vi "TEST-Main.vi"() -> ()   [LabVIEW 2020, in "CSMStand(Lite)-test.lvlib"]
doc: "------------- lvcsm -------------\n[CSMStates]\nItem 0 = \"Event Structure\"\nItem 1 = \"Idle\"\nItem 2 = \"CSM Documentation\"\nItem 3 = \"Error Handler\"\nItem 4 = \"VI Reference\"\nItem 5 = \"Critical Error\"\nItem 6 = \"Target Timeout Error\"\nItem 7 = \"Target Error\"\nItem 8 = \"Async Response\"\nItem 9 = \"Response\"\nItem 10 = \"Async Message Posted\"\nItem 11 = \"Initialize Core Data\"\nItem 12 = \"Exit\"\nItem 13 = \"Data: Initialize\"\nItem 14 = \"Data: Cleanup\"\nItem 15 = \"Events: Register\"\nItem 16 = \"Events: Unregister\"\nItem 17 = \"UI: Initialize\"\nItem 18 = \"UI: Cursor Set\"\nItem 19 = \"UI: Front Panel State\"\nItem 20 = \"Macro: Initialize\"\nItem 21 = \"Macro: Exit\"\nItem 22 = \"API: API1\"\nItem 23 = \"API: API2\"\nItem 24 = \"Internal: action1\"\nItem 25 = \"Internal: action2\"\n\n[CSMStatus]\nItem 0 = \"Error Occurred@Error Handler\""
uses:
  <vilib>/numeric/Random Number (Range) DBL.vi
  510b3246-460f-4579-b188-a02bea6833a2.vi
  <userlib>/_NEVSTOP/Communicable State Machine(CSM)/_Support/Common/Format Timestamp.vi
  <userlib>/_NEVSTOP/Communicable State Machine(CSM)/AdvanceAPI/CSM - Keywords.vi
  <userlib>/_NEVSTOP/Communicable State Machine(CSM)/AdvanceAPI/CSM - Revert Arguments-Safe String.vi
  <userlib>/_NEVSTOP/Communicable State Machine(CSM)/AdvanceAPI/CSM - Compact Multiple States.vi
  <userlib>/_NEVSTOP/Communicable State Machine(CSM)/addons/MassData-Parameter/_support/FGV-MassData(lvlibp).vi
  <userlib>/_NEVSTOP/Communicable State Machine(CSM)/_Shared/Trim Single-line Text.vi
  CSMStand(Lite)-test.lvlib
  <userlib>/_NEVSTOP/Communicable State Machine(CSM)/Communicable State Machine.lvlib
  src/CSMStand(Lite).lvlib
panel:
  in  "TS: Step Complete Handler":bool
  in  "TS: Load Sequence":bool
  out "State History":string
  in  "Init State(\"Macro: Initialize\")":string="Macro: Initialize"
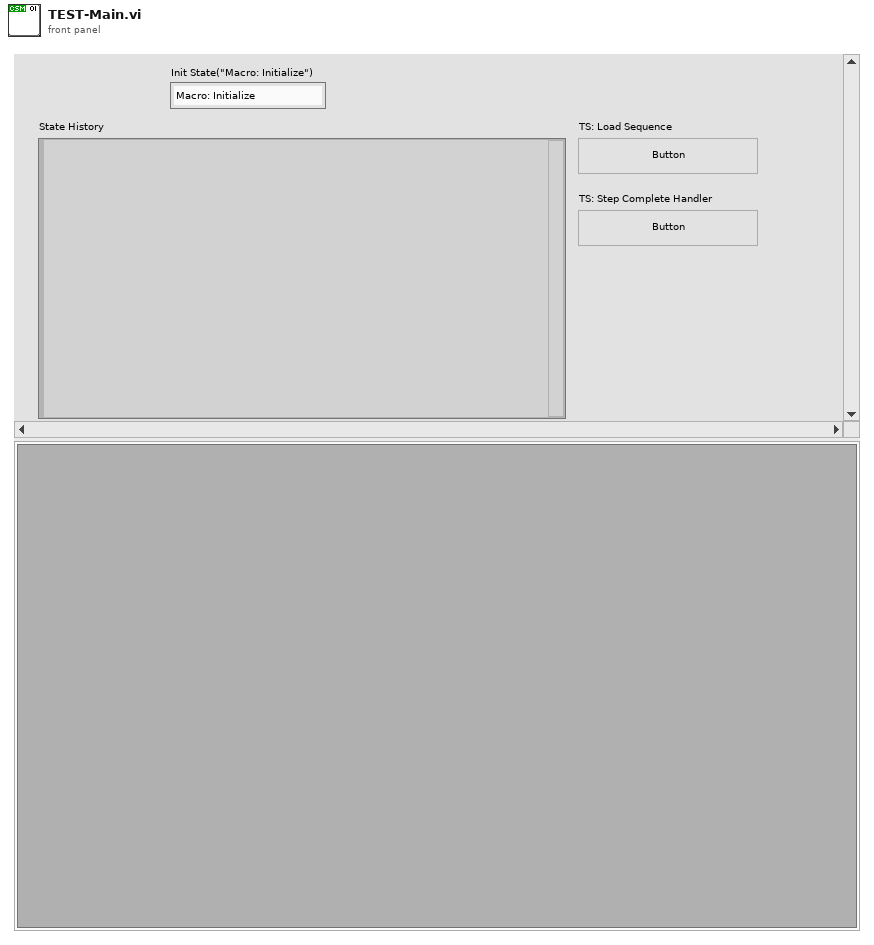
[diagram p1: front panel]
types:
  T1 = enum32{"Invalid", "Standard", "Closed", "Hidden", "Minimized", "Maximized"}
  T2 = enum32{"invalid app kind", "Development System", "Run Time System", "Student Edition", "Embedded LabVIEW", "Evaluation", "Custom"}
  T3 = typedef "Communicable State Machine.lvlib/_CSM_Response Source Message.ctl" = cluster{"‘State":string, "’Arguments":string, "’Error":errorcluster}
  T4 = cluster{i32, string, "error in (no error)":errorcluster}
  T5 = cluster{"Current VI Reference":refnum<vi>, "Close Panel on Exit?":bool}
  T6 = cluster{"Core":cluster{"Current VI Reference":refnum<vi>, "Close Panel on Exit?":bool}, "Your Boolean data":bool, "Sequence":string}
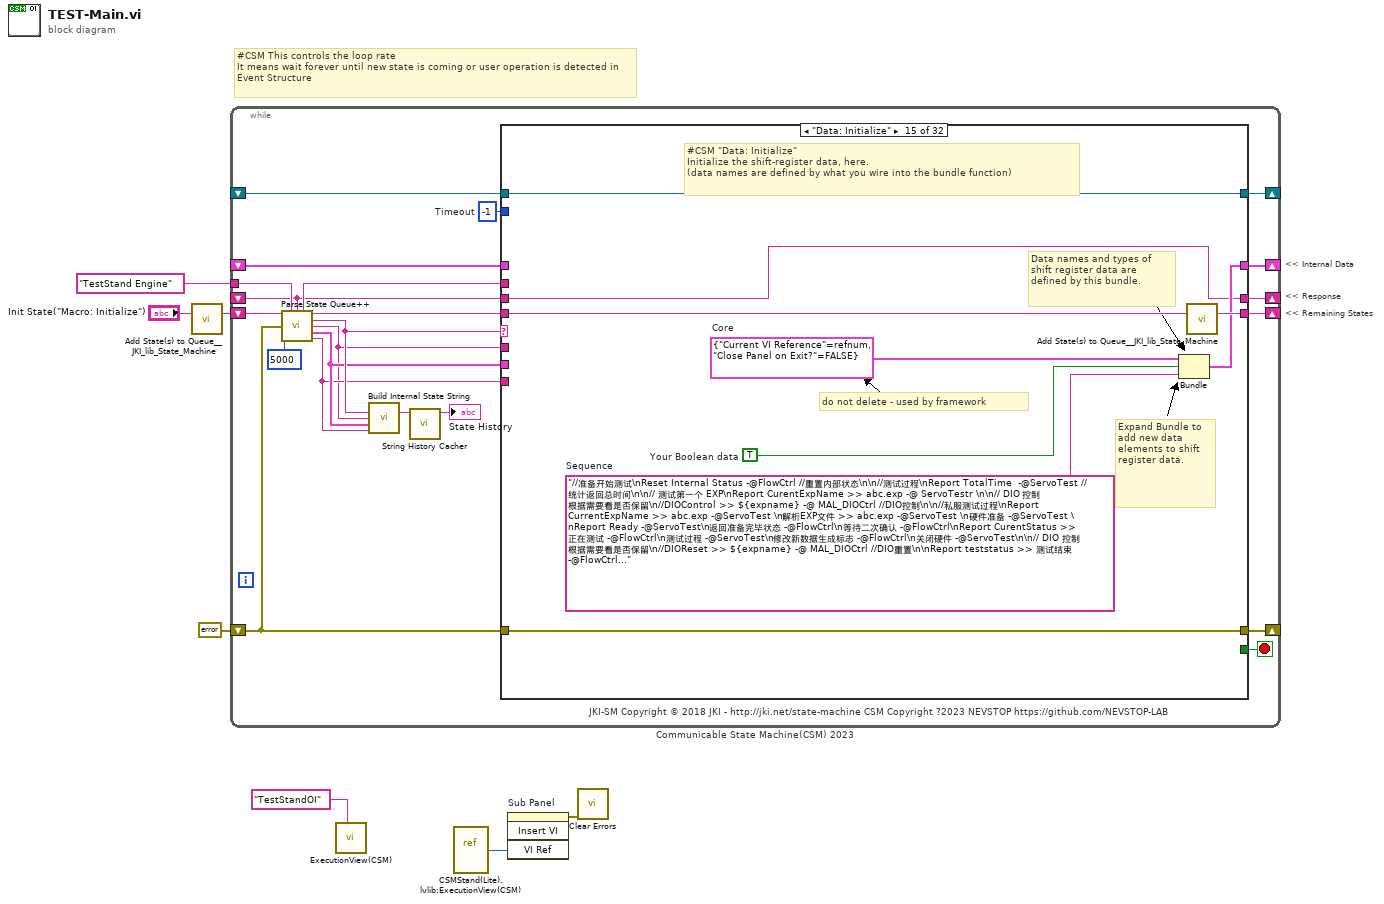
[diagram p0: block diagram]
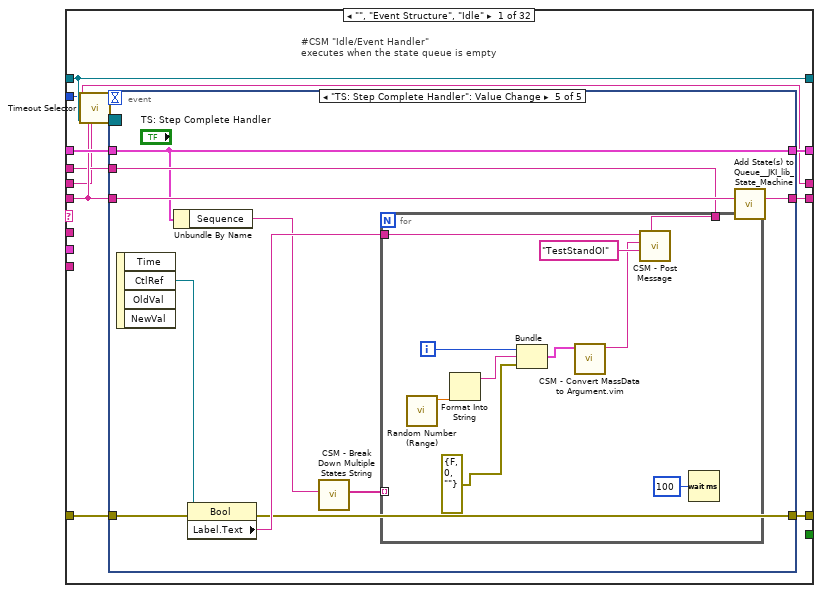
[diagram p2: hidden frame]
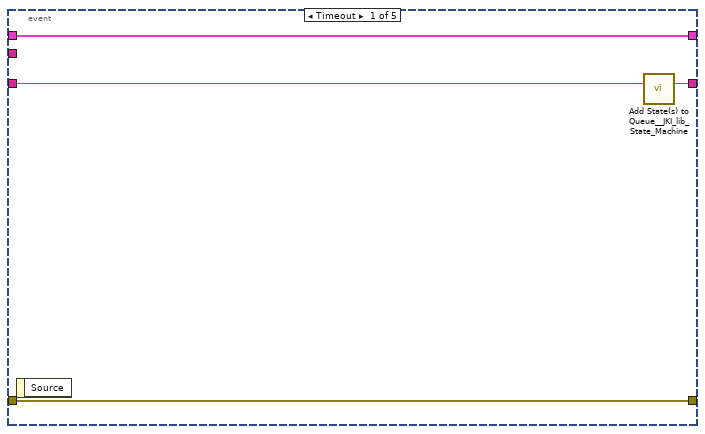
[diagram p3: hidden frame]
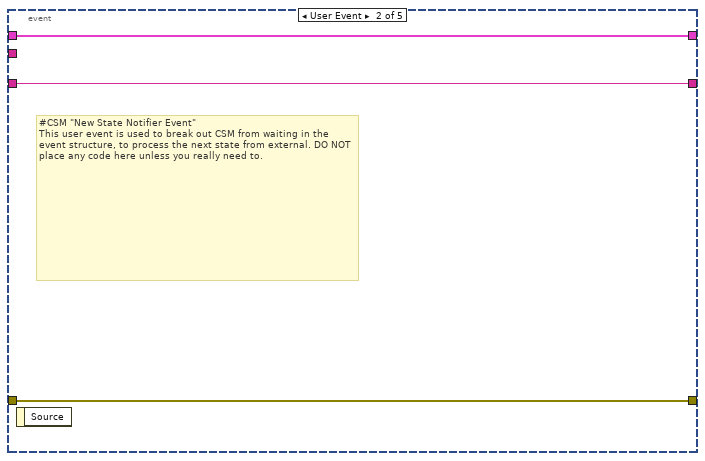
[diagram p4: hidden frame]
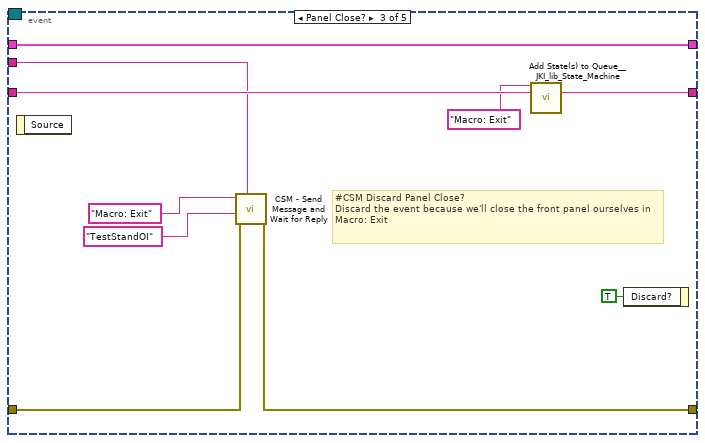
[diagram p5: hidden frame]
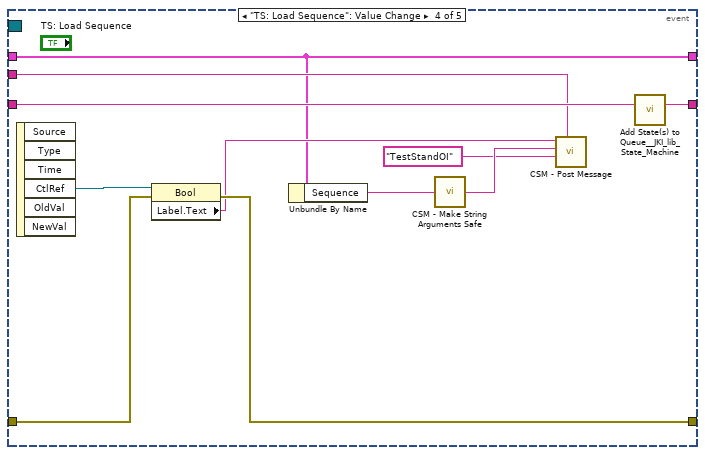
[diagram p6: hidden frame]
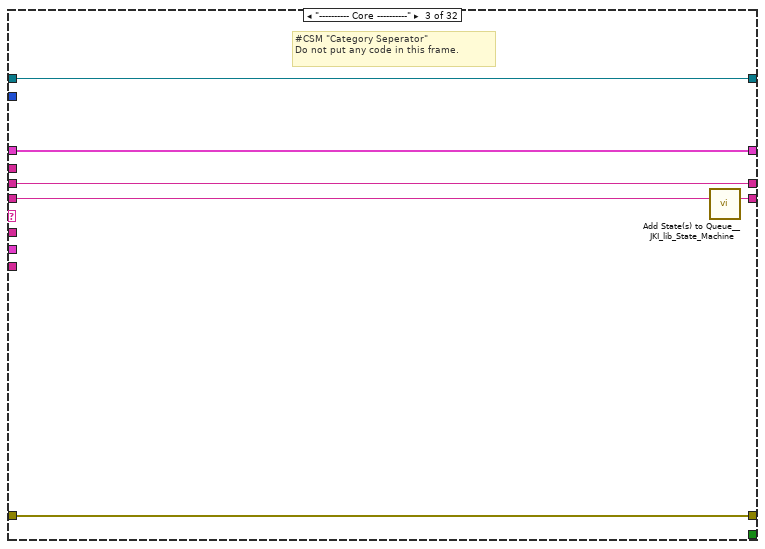
[diagram p8: hidden frame]
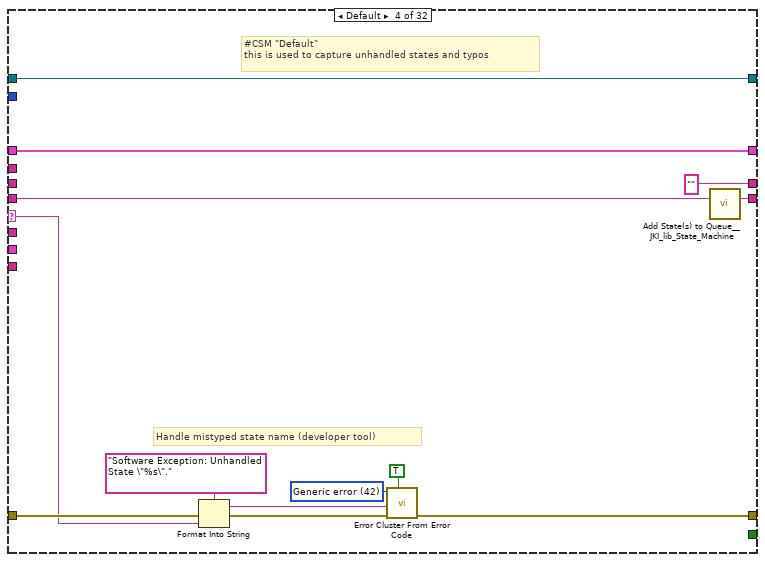
[diagram p9: hidden frame]
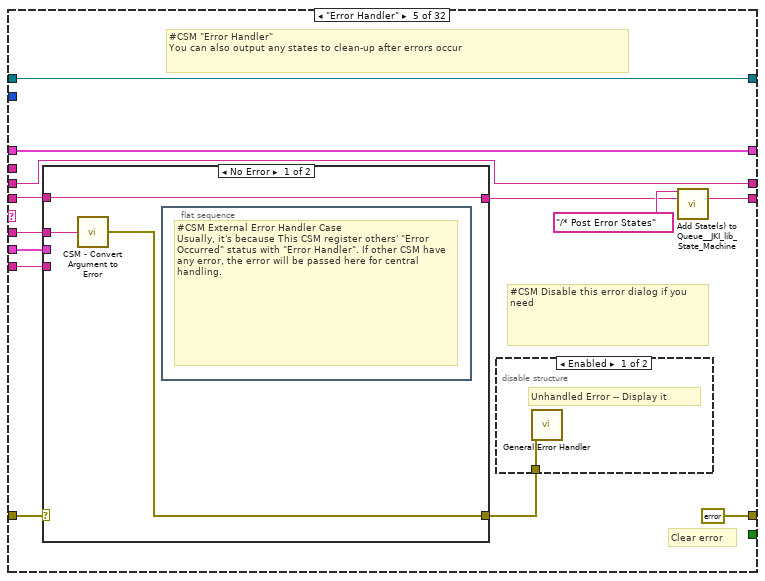
[diagram p10: hidden frame]
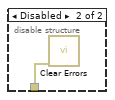
[diagram p11: hidden frame]
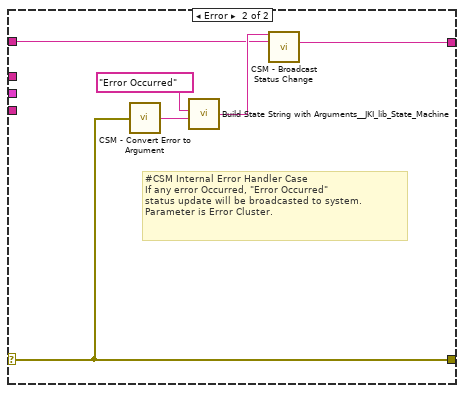
[diagram p12: hidden frame]
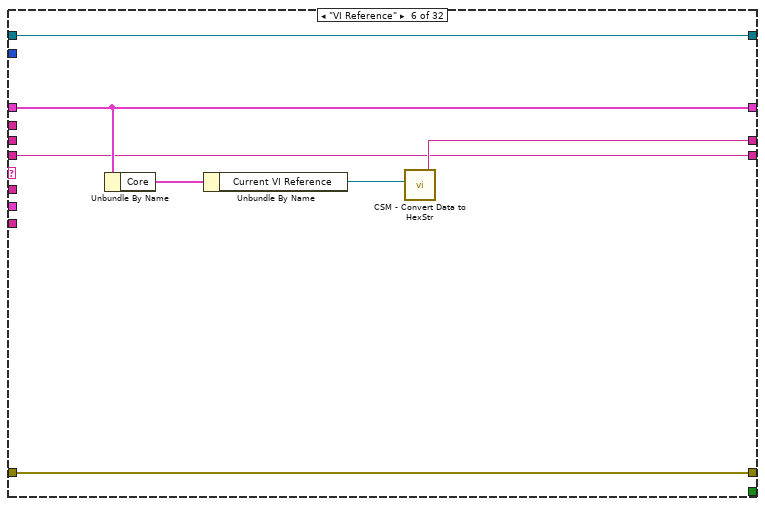
[diagram p13: hidden frame]
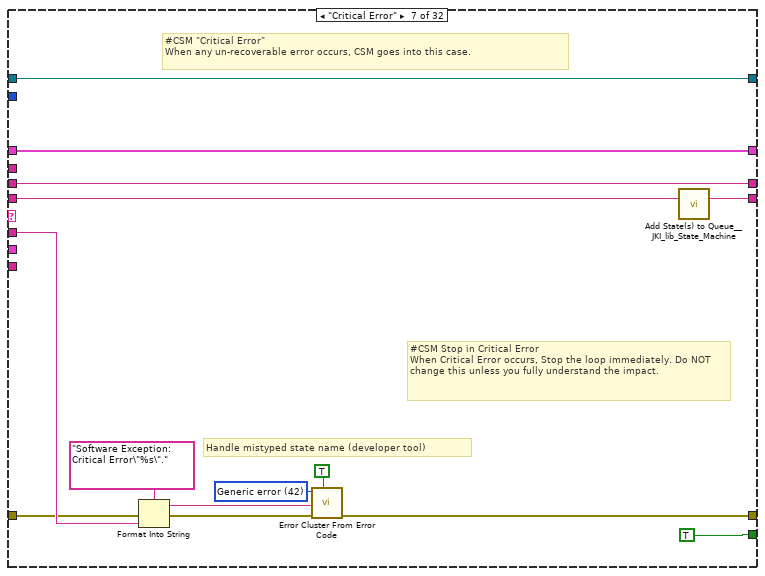
[diagram p14: hidden frame]
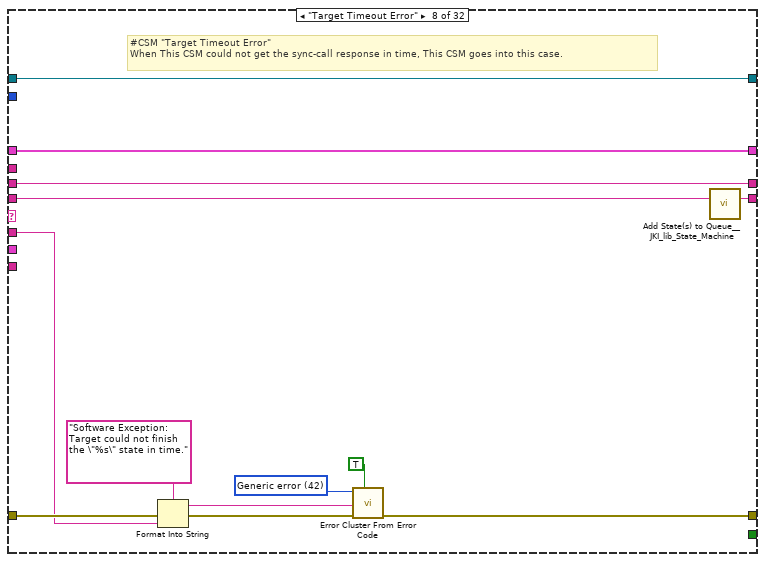
[diagram p15: hidden frame]
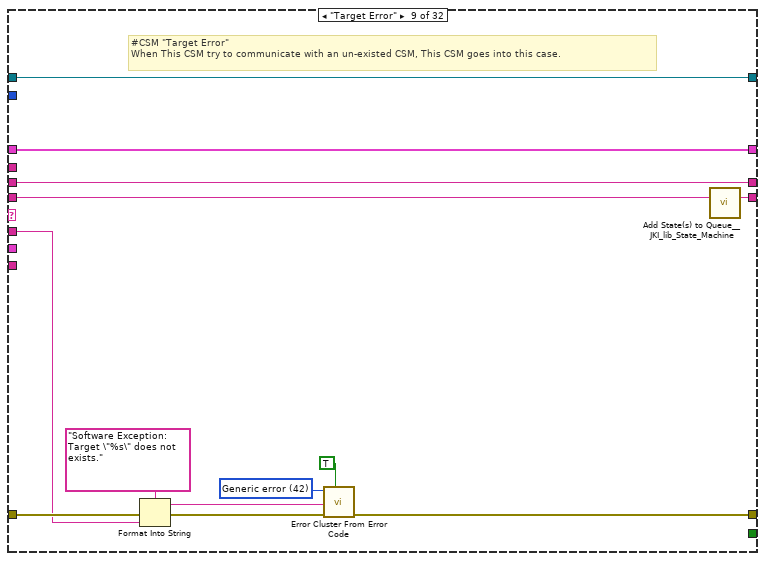
[diagram p16: hidden frame]
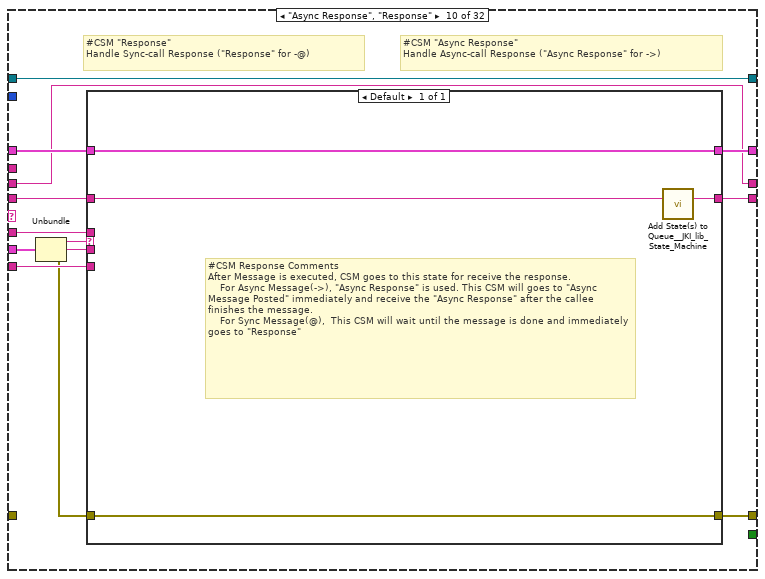
[diagram p17: hidden frame]
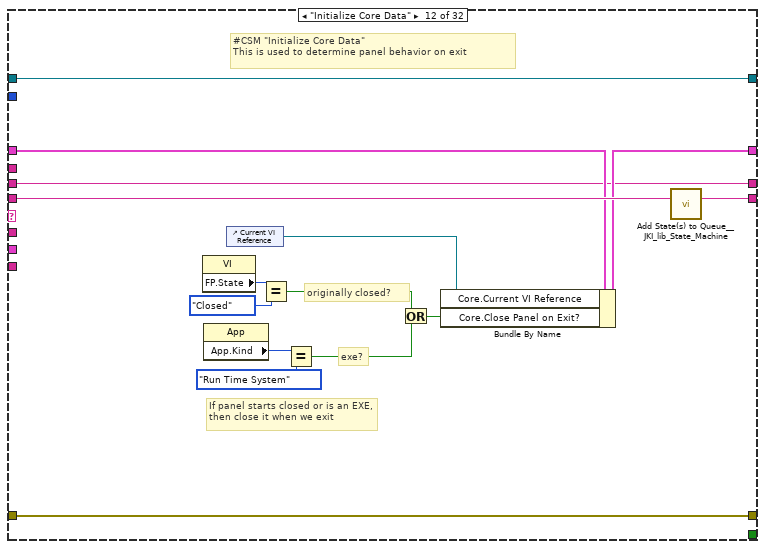
[diagram p19: hidden frame]
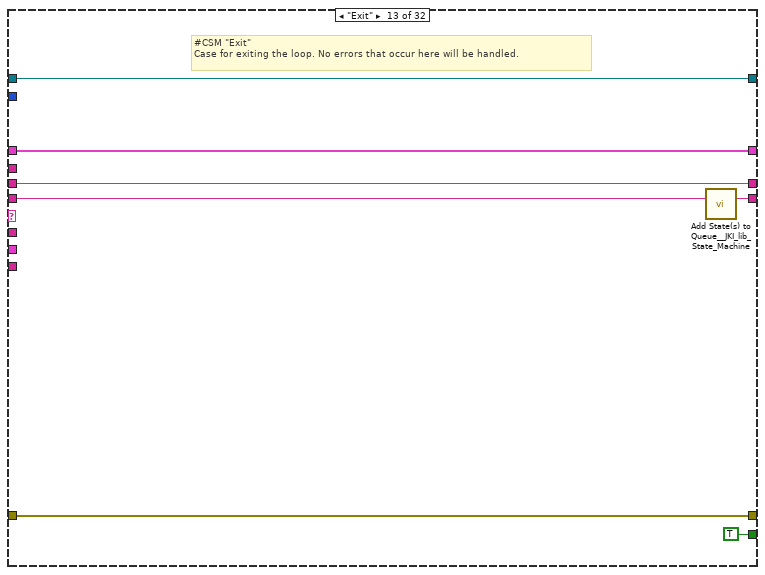
[diagram p20: hidden frame]
diagram:
  # "<< Internal Data"
  # "<< Response"
  # "<< Remaining States"
  # "#CSM This controls the loop rate\nIt means wait forever until new state is coming or user operation is detected in Event Structure"
  n1 = call <vilib>:"Add State(s) to Queue__JKI_lib_State_Machine.vi"("State(s) in (\"\")"="Init State(\"Macro: Initialize\")") -> ("States Out"=w4:string)  [unwired: 14 in]
  n2 = while "Communicable State Machine(CSM) 2023" {
    shift-right: [w24] -> _
    shift-left: _ -> [w23]
    shift-right: [w27] -> _
    shift-left: errorcluster {"status"=FALSE, "code"=0, "source"=""} ("error out") -> [w21]
    shift-right: [w26] -> _
    shift-left: w4 -> [w28]
    tunnel: "TestStand Engine" ("Name(\"\" to use uuid)") -> [w16]
    shift-right: [w19] -> _
    shift-left: _ -> [w9]
    shift-right: [w18] -> _
    shift-left: _ -> [w17]
    stop <- w25 stop-if-true
    w22 = -1  # Timeout
    # "JKI-SM Copyright © 2018 JKI - http://jki.net/state-machine CSM Copyright ?2023 NEVSTOP https://github.com/NEVSTOP-LAB"
    n3 = call <userlib>:"Parse State Queue++.vi"("State Queue"=w28, "Name (\"\" to Use UUID)"=w16, "Response Arguments"=w9, "Previous Error"=w21, "Response Timeout (-2 Use Global Settings)"=5000 ("Response Timeout(1000ms)")) -> ("Name Used"=w10:string, "Remaining States"=w29:string, "Current State"=w13:string, "Arguments"=w8:string, "Additional Information"=w12:T3, "Source CSM"=w11:string)  [unwired: 5 in]
    n4 = call <userlib>:"Build Internal State String.vi"("State"=w13, "Arguments (\"\")"=w8, "Additional Information"=w12, "Source (\"\")"=w11) -> ("State With Arguments"=w14:string)  [unwired: 11 in]
    n5 = call <userlib>:"String History Cacher.vi"("String"=w14) -> ("String Cache"=→"State History":string)  [unwired: 10 in]
    n6 = case shown="\"Data: Initialize\"" w13 {
      selector: w13 -> [_ _ _ w102 _ _ _ _ _ _ _ _ _ _ _ _ _ _ _ _ _ _ _ _ _ _ _ _ _ _ _ _]
      tunnel: w29 -> [w32 w93 w99 w106 w118 w138 w156 w165 w178 w194 w204 w220 w227 w233 w242 w250 w256 w264 w269 w276 w282 w290 w307 w378 w385 w398 w402 w407 w412 w419 w425 w431]
      tunnel: w8 -> [_ _ _ _ w116 _ w149 w161 w174 w188 _ _ _ _ _ _ _ _ _ _ _ w285 w301 _ _ _ _ _ _ _ _ _]
      tunnel: w23 -> [w39 w92 w96 w104 w124 w143 w157 w163 w176 w192 w203 w213 w225 w230 _ w245 w253 w263 w268 w273 w280 w288 w303 w375 w382 w395 w401 w406 w411 w416 w422 w428]
      tunnel: [w38 w91 w97 w108 errorcluster {"status"=FALSE, "code"=0, "source"=""} ("error out") w137 w145 w159 w172 w191 w205 w217 w224 w231 w239 w246 w254 w258 w267 w274 w279 w286 w304 w376 w383 w396 w403 w408 w413 w417 w423 w429] -> w27
      tunnel: w21 -> [w37 w91 w97 w107 w122 w137 w146 w166 w179 _ w205 w217 w224 w231 w239 w247 w254 _ w270 w274 w279 w287 w305 w376 w383 w396 w403 w408 w413 w417 w423 w429]
      tunnel: [w40 w93 w98 w105 w120 w138 w155 w164 w177 w195 w204 w219 w226 w232 w241 w249 w255 w264 w269 w275 w281 w289 w306 w377 w384 w397 w402 w407 w412 w418 w424 w430] -> w26
      tunnel: [_ _ _ _ _ _ TRUE _ _ _ _ _ TRUE _ _ _ _ _ _ _ _ _ _ _ _ _ _ _ _ _ _ _] -> w25
      tunnel: [w36 w92 w96 w104 w124 w143 w157 w163 w176 w193 w203 w218 w225 w230 w240 w245 w253 w263 w268 w273 w280 w288 w303 w375 w382 w395 w401 w406 w411 w416 w422 w428] -> w24
      tunnel: w22 -> [w34 _ _ _ _ _ _ _ _ _ _ _ _ _ _ _ _ _ _ _ _ _ _ _ _ _ _ _ _ _ _ _]
      tunnel: w11 -> [_ _ _ _ w115 _ _ _ _ w189 _ _ _ _ _ _ _ _ _ _ _ _ _ _ _ _ _ _ _ _ _ _]
      tunnel: w12 -> [_ _ _ _ w114 _ _ _ _ w190 _ _ _ _ _ _ _ _ _ _ _ _ _ _ _ _ _ _ _ _ _ _]
      tunnel: [w30 w89 w94 "" w113 w140 w144 w158 w171 w184 w201 w206 w221 w228 w234 w243 w251 w257 w265 w271 w277 w283 w299 w373 w379 w386 w399 "API1 Response" w409 w414 w420 w426] -> w19
      tunnel: [w35 w90 w95 w100 w123 w139 w147 w160 w173 w196 w202 w207 w222 w229 w236 w244 w252 w262 w266 w272 w278 w284 w300 w374 w380 w388 w400 w405 w410 w415 w421 w427] -> w18
      tunnel: w17 -> [w35 w90 w95 w100 w123 w139 w147 w160 w173 w196 w202 w207 w222 w229 w236 w244 w252 _ w266 w272 w278 w284 w300 w374 w380 w388 w400 w405 w410 w415 w421 w427]
      tunnel: w10 -> [w31 _ _ _ _ _ _ _ _ _ _ _ _ _ _ _ _ w261 _ _ _ _ _ _ _ _ _ _ _ _ _ _]
      tunnel: w9 -> [w30 w89 w94 _ w113 _ w144 w158 w171 w184 w201 w206 w221 w228 w234 w243 w251 w257 w265 w271 w277 w283 w299 w373 w379 w386 w399 _ w409 w414 w420 w426]
      frame "", "Event Structure", "Idle" {
        # "#CSM \"Idle/Event Handler\"\nexecutes when the state queue is empty"
        n7 = call <userlib>:"Timeout Selector.vi"("Remaining States"=w32, "Timeout Expected"=w34) -> ("Timeout"=w33:i32)  [unwired: 5 in]
        n8 = event shown="[4] \"TS: Step Complete Handler\": Value Change" {
          selector: w35 -> [_ _ _ _ _]
          dyn-events: _ -> [_ _ _ _ _]
          timeout: w33 -> [_ _ _ _ _]
          tunnel: w32 -> [w44 w46 w57 w65 w76]
          tunnel: [w43 w46 w56 w64 w75] -> w40
          tunnel: w39 -> [w41 w47 w55 w59 w72]
          tunnel: [w42 w45 w51 w66 w69] -> w38
          tunnel: w37 -> [w42 w45 w52 w67 w77]
          tunnel: [w41 w47 w55 w59 w72] -> w36
          tunnel: w31 -> [_ _ w50 w63 w74]
          event Timeout {
            n9 = event-data() -> ()  [unwired: 1 in, 1 out]
            n10 = call <vilib>:"Add State(s) to Queue__JKI_lib_State_Machine.vi"("State(s) in (\"\")"=w44) -> ("States Out"=w43:string)  [unwired: 14 in]
          }
          event User Event {
            # "#CSM \"New State Notifier Event\"\nThis user event is used to break out CSM from waiting in the event structure, to process the next state from external. DO NOT place any code here unless you really need to."
            n11 = event-data() -> ()  [unwired: 1 in, 1 out]
          }
          event Panel Close? {
            # "#CSM Discard Panel Close?\nDiscard the event because we'll close the front panel ourselves in Macro: Exit"
            n12 = event-data() -> ()  [unwired: 1 in, 1 out]
            n13 = call <userlib>:"CSM - Send Message and Wait for Reply.vi"("Current Module (\"\" to Generate an ID)"=w50, "Error In (No Error)"=w52, "Target Module"="TestStandOI", "State"="Macro: Exit" ("Target Module")) -> ("error out"=w51:errorcluster)  [unwired: 5 in, 2 out]
            n14 = call <vilib>:"Add State(s) to Queue__JKI_lib_State_Machine.vi"("State(s) in Front (\"\")"="Macro: Exit", "State(s) in (\"\")"=w57) -> ("States Out"=w56:string)  [unwired: 13 in]
            n15 = event-data("Discard?"=TRUE) -> ()  [unwired: 1 in, 1 out]
          }
          event "TS: Load Sequence": Value Change {
            n16 = event-data() -> ("CtlRef"=w68:refnum<vi>)  [unwired: 1 in, 5 out]
            n17 = property class="Bool"(reference=w68, error in=w67) -> (error out=w66:errorcluster, "Label.Text"=w60:string)  [unwired: 1 out]
            n18 = Unbundle By Name(w59) -> ("Sequence"=w58:string)
            n19 = call <userlib>:"CSM - Make String Arguments Safe.vi"("Argument String"=w58) -> ("Safe Argument String"=w62:string)  [unwired: 8 in]
            n20 = call <userlib>:"CSM - Post Message.vi"("Current Module (\"\" to Generate an ID)"=w63, "Target Module"="TestStandOI", "Arguments (\"\")"=w62, "State"=w60) -> ()  [unwired: 7 in, 1 out]
            n21 = call <vilib>:"Add State(s) to Queue__JKI_lib_State_Machine.vi"("State(s) in (\"\")"=w65) -> ("States Out"=w64:string)  [unwired: 14 in]
          }
          event "TS: Step Complete Handler": Value Change {
            n22 = event-data() -> ("CtlRef"=w78:refnum<vi>)  [unwired: 1 in, 3 out]
            n23 = Unbundle By Name(w72) -> ("Sequence"=w71:string)
            n24 = property class="Bool"(reference=w78, error in=w77) -> (error out=w69:errorcluster, "Label.Text"=w73:string)  [unwired: 1 out]
            n25 = call <userlib>:"CSM - Break Down Multiple States String.vi"("States"=w71) -> ("Multiple States"=w70:string[])  [unwired: 10 in]
            n26 = for {
              tunnel: w74 -> [w88]
              tunnel: w73 -> [w86]
              tunnel: w70 -> [_] mode=indexing
              i -> [w85]
              n27 = call-poly <vilib>:"Random Number (Range).vi"() -> ("number"=w82:dbl)  [unwired: 11 in]
              n28 = Format Into String(w82) -> (resulting string=w81:string)  [unwired: 3 in, 1 out]
              n29 = Bundle(w85, w81, "error in (no error)"=errorcluster {"status"=FALSE, "code"=0, "source"=""}) -> (w79:T4)  [unwired: 1 in]
              n30 = call "CSM - Convert MassData to Argument.vim"("Data"=w79) -> ("MassData Argument"=w80:string)  [unwired: 7 in, 1 out]
              n31 = call <userlib>:"CSM - Post Message.vi"("Current Module (\"\" to Generate an ID)"=w88, "Target Module"="TestStandOI", "Arguments (\"\")"=w80, "State"=w86) -> ()  [unwired: 7 in, 1 out]
              n32 = Wait (ms)(milliseconds to wait=u32 100) -> ()  [unwired: 1 out]
            }
            n33 = call <vilib>:"Add State(s) to Queue__JKI_lib_State_Machine.vi"("State(s) in (\"\")"=w76) -> ("States Out"=w75:string)  [unwired: 14 in]
          }
        }
      }
      frame "CSM Documentation" {
        # "#CSM \"Documentation\"\nCase for holding CSM Documenation"
      }
      frame "---------- Core ----------" {
        # "#CSM \"Category Seperator\"\nDo not put any code in this frame."
        n34 = call <vilib>:"Add State(s) to Queue__JKI_lib_State_Machine.vi"("State(s) in (\"\")"=w99) -> ("States Out"=w98:string)  [unwired: 14 in]
      }
      frame Default {
        w111 = 42 items=["No error", "Argument error", "Memory is full", "Out of zone", "End of file", "File already open", "Generic file I/O error", "File not found", "File permission error", "Disk is full", "Duplicate path", "Too many files open", "System feature not enabled", "Resource file not found", "Cannot add resource", "Resource not found", "Image not found", "Image memory error", "Pen does not exist", "Config type invalid", "Config token not found", "Config parse error", "Config memory error", "Bad external code format", "Bad external code offset", "External code not present", "Null window", "Destroy window error", "Null menu", "Print aborted", "Bad print record", "Print driver error", "Windows error during printing", "Memory error during printing", "Print dialog error", "Generic print error", "Invalid device refnum", "Device not found", "Device parameter error", "Device unit error", "Cannot open device", "Device call aborted", "Generic error", "Cancelled by user", "Object ID too low", "Object ID too high", "Object not in heap", "Unknown heap", "Unknown object (invalid DefProc)", "Unknown object (DefProc not in table)", "Message out of range", "Invalid (null) method", "Unknown message", "Manager call not supported", "Bad address", "Network operation in progress", "Network operation timed out", "Connection is busy", "Network attribute not supported", "Network error", "Address in use", "System out of memory", "Connection aborted", "Connection refused", "Not connected", "Already connected", "Connection closed", "Initialization error (interapplication manager)", "Bad occurrence", "Wait on unbound occurrence handler", "Occurrence queue overflow", "Datalog type conflict", "Unused", "Unrecognized type (interapplication manager)", "Memory corrupt", "Failed to make temporary DLL", "Old CIN version", "Drag socket not found", "Failed to load drop-object", "Failed to register OLE object", "Failed to release OLE object", "Format specifier type mismatch", "Unknown format specifier", "Too few format specifiers", "Too many format specifiers", "Scan failed", "Newer CIN version", "Error converting to variant", "Runtime menu error", "Password tampered", "Variant attribute not found", "Incompatible variant data type", "Event data is not available", "Event Store is not present", "Occurrence is not found", "Event Queue is not created", "Event info is not available", "Refnum passed is NULL", "Error retrieving Class GUID", "Error retrieving CoClass GUID", "Error retrieving TypeLib GUID.", "Bad built application magic bytes.", "Specific driver is different from the specific driver associated with the Logical Name.", "There is no session opened to the class driver.", "Max Error", "MAX - Error with config objects", "MAX - Error loading configuration", "MAX - Group not supported"]
        # "#CSM \"Default\"\nthis is used to capture unhandled states and typos"
        # "Handle mistyped state name (developer tool)"
        n35 = Format Into String(format string="Software Exception: Unhandled State \"%s\"." ("message"), error in=w107, w102) -> (resulting string=w110:string, error out=w109:errorcluster)  [unwired: 1 in]
        n36 = call <vilib>:"Error Cluster From Error Code.vi"("show call chain? (False)"=TRUE, "error in (no error)"=w109, "error message (\"\")"=w110, "error code (0)"=w111) -> ("error out"=w108:errorcluster)  [unwired: 5 in]
        n37 = call <vilib>:"Add State(s) to Queue__JKI_lib_State_Machine.vi"("State(s) in (\"\")"=w106) -> ("States Out"=w105:string)  [unwired: 14 in]
      }
      frame "Error Handler" {
        # "#CSM Disable this error dialog if you need"
        # "#CSM \"Error Handler\"\nYou can also output any states to clean-up after errors occur"
        # "Clear error"
        n38 = case shown="No Error" w122 {
          selector: w122 -> [_ w131]
          tunnel: [w129 w133] -> w119
          tunnel: w118 -> [w129 w132]
          tunnel: [w128 w131] -> w117
          tunnel: w116 -> [w130 _]
          tunnel: w115 -> [_ _]
          tunnel: w114 -> [_ _]
          frame No Error {
            n39 = call <userlib>:"CSM - Convert Argument to Error.vi"("Argument"=w130) -> ("Error"=w128:errorcluster)  [unwired: 4 in]
            n40 = flat-sequence {
              frame #0 {
                # "#CSM External Error Handler Case\nUsually, it's because This CSM register others' \"Error Occurred\" status with \"Error Handler\". If other CSM have any error, the error will be passed here for central handling."
              }
            }
          }
          frame Error {
            # "#CSM Internal Error Handler Case \nIf any error Occurred, \"Error Occurred\" \nstatus update will be broadcasted to system.\nParameter is Error Cluster."
            n41 = call <userlib>:"CSM - Convert Error to Argument.vi"("Error"=w131) -> ("Argument"=w135:string)  [unwired: 4 in]
            n42 = call <vilib>:"Build State String with Arguments__JKI_lib_State_Machine.vi"("Arguments (\"\")"=w135, "State"="Error Occurred" ("Status with Arguments")) -> ("State with Arguments"=w134:string)  [unwired: 4 in]
            n43 = call <userlib>:"CSM - Broadcast Status Change.vi"("Status With Arguments"=w134, "State Queue"=w132) -> ("Remaining States"=w133:string)  [unwired: 13 in]
          }
        }
        n44 = disable-structure shown="Enabled" {
          disable-tunnel: w117 -> [w126 w127]
          frame Enabled {
            # "Unhandled Error -- Display it"
            n45 = call <vilib>:"General Error Handler.vi"("error in (no error)"=w126) -> ()  [unwired: 10 in, 5 out]
          }
          frame Disabled {
            n46 = call <vilib>:"Clear Errors.vi"("error in (no error)"=w127) -> ()  [unwired: 5 in, 2 out]
          }
        }
        n47 = call <vilib>:"Add State(s) to Queue__JKI_lib_State_Machine.vi"("State(s) in Front (\"\")"="/* Post Error States", "State(s) in (\"\")"=w119) -> ("States Out"=w120:string)  [unwired: 13 in]
      }
      frame "VI Reference" {
        n48 = Unbundle By Name(w143) -> ("Core"=w142:T5)
        n49 = Unbundle By Name(w142) -> ("Current VI Reference"=w141:refnum<vi>)
        n50 = call <userlib>:"CSM - Convert Data to HexStr.vi"("Variant"=w141) -> ("HEX String (0-9,A-F)"=w140:string)  [unwired: 8 in]
      }
      frame "Critical Error" {
        w153 = 42 items=["No error", "Argument error", "Memory is full", "Out of zone", "End of file", "File already open", "Generic file I/O error", "File not found", "File permission error", "Disk is full", "Duplicate path", "Too many files open", "System feature not enabled", "Resource file not found", "Cannot add resource", "Resource not found", "Image not found", "Image memory error", "Pen does not exist", "Config type invalid", "Config token not found", "Config parse error", "Config memory error", "Bad external code format", "Bad external code offset", "External code not present", "Null window", "Destroy window error", "Null menu", "Print aborted", "Bad print record", "Print driver error", "Windows error during printing", "Memory error during printing", "Print dialog error", "Generic print error", "Invalid device refnum", "Device not found", "Device parameter error", "Device unit error", "Cannot open device", "Device call aborted", "Generic error", "Cancelled by user", "Object ID too low", "Object ID too high", "Object not in heap", "Unknown heap", "Unknown object (invalid DefProc)", "Unknown object (DefProc not in table)", "Message out of range", "Invalid (null) method", "Unknown message", "Manager call not supported", "Bad address", "Network operation in progress", "Network operation timed out", "Connection is busy", "Network attribute not supported", "Network error", "Address in use", "System out of memory", "Connection aborted", "Connection refused", "Not connected", "Already connected", "Connection closed", "Initialization error (interapplication manager)", "Bad occurrence", "Wait on unbound occurrence handler", "Occurrence queue overflow", "Datalog type conflict", "Unused", "Unrecognized type (interapplication manager)", "Memory corrupt", "Failed to make temporary DLL", "Old CIN version", "Drag socket not found", "Failed to load drop-object", "Failed to register OLE object", "Failed to release OLE object", "Format specifier type mismatch", "Unknown format specifier", "Too few format specifiers", "Too many format specifiers", "Scan failed", "Newer CIN version", "Error converting to variant", "Runtime menu error", "Password tampered", "Variant attribute not found", "Incompatible variant data type", "Event data is not available", "Event Store is not present", "Occurrence is not found", "Event Queue is not created", "Event info is not available", "Refnum passed is NULL", "Error retrieving Class GUID", "Error retrieving CoClass GUID", "Error retrieving TypeLib GUID.", "Bad built application magic bytes.", "Specific driver is different from the specific driver associated with the Logical Name.", "There is no session opened to the class driver.", "Max Error", "MAX - Error with config objects", "MAX - Error loading configuration", "MAX - Group not supported"]
        # "#CSM \"Critical Error\"\nWhen any un-recoverable error occurs, CSM goes into this case."
        # "#CSM Stop in Critical Error\nWhen Critical Error occurs, Stop the loop immediately. Do NOT change this unless you fully understand the impact."
        # "Handle mistyped state name (developer tool)"
        n51 = Format Into String(format string="Software Exception: Critical Error\"%s\"." ("message"), error in=w146, w149) -> (resulting string=w152:string, error out=w151:errorcluster)  [unwired: 1 in]
        n52 = call <vilib>:"Error Cluster From Error Code.vi"("show call chain? (False)"=TRUE, "error in (no error)"=w151, "error message (\"\")"=w152, "error code (0)"=w153) -> ("error out"=w145:errorcluster)  [unwired: 5 in]
        n53 = call <vilib>:"Add State(s) to Queue__JKI_lib_State_Machine.vi"("State(s) in (\"\")"=w156) -> ("States Out"=w155:string)  [unwired: 14 in]
      }
      frame "Target Timeout Error" {
        w169 = 42 items=["No error", "Argument error", "Memory is full", "Out of zone", "End of file", "File already open", "Generic file I/O error", "File not found", "File permission error", "Disk is full", "Duplicate path", "Too many files open", "System feature not enabled", "Resource file not found", "Cannot add resource", "Resource not found", "Image not found", "Image memory error", "Pen does not exist", "Config type invalid", "Config token not found", "Config parse error", "Config memory error", "Bad external code format", "Bad external code offset", "External code not present", "Null window", "Destroy window error", "Null menu", "Print aborted", "Bad print record", "Print driver error", "Windows error during printing", "Memory error during printing", "Print dialog error", "Generic print error", "Invalid device refnum", "Device not found", "Device parameter error", "Device unit error", "Cannot open device", "Device call aborted", "Generic error", "Cancelled by user", "Object ID too low", "Object ID too high", "Object not in heap", "Unknown heap", "Unknown object (invalid DefProc)", "Unknown object (DefProc not in table)", "Message out of range", "Invalid (null) method", "Unknown message", "Manager call not supported", "Bad address", "Network operation in progress", "Network operation timed out", "Connection is busy", "Network attribute not supported", "Network error", "Address in use", "System out of memory", "Connection aborted", "Connection refused", "Not connected", "Already connected", "Connection closed", "Initialization error (interapplication manager)", "Bad occurrence", "Wait on unbound occurrence handler", "Occurrence queue overflow", "Datalog type conflict", "Unused", "Unrecognized type (interapplication manager)", "Memory corrupt", "Failed to make temporary DLL", "Old CIN version", "Drag socket not found", "Failed to load drop-object", "Failed to register OLE object", "Failed to release OLE object", "Format specifier type mismatch", "Unknown format specifier", "Too few format specifiers", "Too many format specifiers", "Scan failed", "Newer CIN version", "Error converting to variant", "Runtime menu error", "Password tampered", "Variant attribute not found", "Incompatible variant data type", "Event data is not available", "Event Store is not present", "Occurrence is not found", "Event Queue is not created", "Event info is not available", "Refnum passed is NULL", "Error retrieving Class GUID", "Error retrieving CoClass GUID", "Error retrieving TypeLib GUID.", "Bad built application magic bytes.", "Specific driver is different from the specific driver associated with the Logical Name.", "There is no session opened to the class driver.", "Max Error", "MAX - Error with config objects", "MAX - Error loading configuration", "MAX - Group not supported"]
        # "#CSM \"Target Timeout Error\"\nWhen This CSM could not get the sync-call response in time, This CSM goes into this case."
        n54 = Format Into String(format string="Software Exception: Target could not finish the \"%s\" state in time." ("message"), error in=w166, w161) -> (resulting string=w168:string, error out=w167:errorcluster)  [unwired: 1 in]
        n55 = call <vilib>:"Error Cluster From Error Code.vi"("show call chain? (False)"=TRUE, "error in (no error)"=w167, "error message (\"\")"=w168, "error code (0)"=w169) -> ("error out"=w159:errorcluster)  [unwired: 5 in]
        n56 = call <vilib>:"Add State(s) to Queue__JKI_lib_State_Machine.vi"("State(s) in (\"\")"=w165) -> ("States Out"=w164:string)  [unwired: 14 in]
      }
      frame "Target Error" {
        w182 = 42 items=["No error", "Argument error", "Memory is full", "Out of zone", "End of file", "File already open", "Generic file I/O error", "File not found", "File permission error", "Disk is full", "Duplicate path", "Too many files open", "System feature not enabled", "Resource file not found", "Cannot add resource", "Resource not found", "Image not found", "Image memory error", "Pen does not exist", "Config type invalid", "Config token not found", "Config parse error", "Config memory error", "Bad external code format", "Bad external code offset", "External code not present", "Null window", "Destroy window error", "Null menu", "Print aborted", "Bad print record", "Print driver error", "Windows error during printing", "Memory error during printing", "Print dialog error", "Generic print error", "Invalid device refnum", "Device not found", "Device parameter error", "Device unit error", "Cannot open device", "Device call aborted", "Generic error", "Cancelled by user", "Object ID too low", "Object ID too high", "Object not in heap", "Unknown heap", "Unknown object (invalid DefProc)", "Unknown object (DefProc not in table)", "Message out of range", "Invalid (null) method", "Unknown message", "Manager call not supported", "Bad address", "Network operation in progress", "Network operation timed out", "Connection is busy", "Network attribute not supported", "Network error", "Address in use", "System out of memory", "Connection aborted", "Connection refused", "Not connected", "Already connected", "Connection closed", "Initialization error (interapplication manager)", "Bad occurrence", "Wait on unbound occurrence handler", "Occurrence queue overflow", "Datalog type conflict", "Unused", "Unrecognized type (interapplication manager)", "Memory corrupt", "Failed to make temporary DLL", "Old CIN version", "Drag socket not found", "Failed to load drop-object", "Failed to register OLE object", "Failed to release OLE object", "Format specifier type mismatch", "Unknown format specifier", "Too few format specifiers", "Too many format specifiers", "Scan failed", "Newer CIN version", "Error converting to variant", "Runtime menu error", "Password tampered", "Variant attribute not found", "Incompatible variant data type", "Event data is not available", "Event Store is not present", "Occurrence is not found", "Event Queue is not created", "Event info is not available", "Refnum passed is NULL", "Error retrieving Class GUID", "Error retrieving CoClass GUID", "Error retrieving TypeLib GUID.", "Bad built application magic bytes.", "Specific driver is different from the specific driver associated with the Logical Name.", "There is no session opened to the class driver.", "Max Error", "MAX - Error with config objects", "MAX - Error loading configuration", "MAX - Group not supported"]
        # "#CSM \"Target Error\"\nWhen This CSM try to communicate with an un-existed CSM, This CSM goes into this case."
        n57 = Format Into String(format string="Software Exception: Target \"%s\" does not exists." ("message"), error in=w179, w174) -> (resulting string=w181:string, error out=w180:errorcluster)  [unwired: 1 in]
        n58 = call <vilib>:"Error Cluster From Error Code.vi"("show call chain? (False)"=TRUE, "error in (no error)"=w180, "error message (\"\")"=w181, "error code (0)"=w182) -> ("error out"=w172:errorcluster)  [unwired: 5 in]
        n59 = call <vilib>:"Add State(s) to Queue__JKI_lib_State_Machine.vi"("State(s) in (\"\")"=w178) -> ("States Out"=w177:string)  [unwired: 14 in]
      }
      frame "Async Response", "Response" {
        # "#CSM \"Async Response\"\nHandle Async-call Response (\"Async Response\" for ->)"
        # "#CSM \"Response\"\nHandle Sync-call Response (\"Response\" for -@)"
        n60 = Unbundle(w190) -> ("‘State"=w187:string, "’Arguments"=w186:string, "’Error"=w185:errorcluster)
        n61 = case shown="Default" w187 {
          tunnel: [w197] -> w195
          tunnel: w194 -> [w198]
          tunnel: [w200] -> w193
          tunnel: w192 -> [w200]
          tunnel: [w199] -> w191
          tunnel: w185 -> [w199]
          tunnel: w189 -> [_]
          tunnel: w188 -> [_]
          tunnel: w186 -> [_]
          frame Default {
            # "#CSM Response Comments\nAfter Message is executed, CSM goes to this state for receive the response.\n    For Async Message(->), \"Async Response\" is used. This CSM will goes to \"Async Message Posted\" immediately and receive the \"Async Response\" after the callee finishes the message.\n    For Sync Message(@),  This CSM will wait until the message is done and immediately goes to \"Response\""
            n62 = call <vilib>:"Add State(s) to Queue__JKI_lib_State_Machine.vi"("State(s) in (\"\")"=w198) -> ("States Out"=w197:string)  [unwired: 14 in]
          }
        }
      }
      frame "Async Message Posted" {
        # "#CSM \"Async Message Posted\"\nAfter Async Message is posted (-> or ->| ), CSM goes to this state for post-action.\nYou can use Argument - State to tell which Async Message is called."
      }
      frame "Initialize Core Data" {
        # "#CSM \"Initialize Core Data\"\nThis is used to determine panel behavior on exit"
        # "originally closed?"
        # "exe?"
        # "If panel starts closed or is an EXE, then close it when we exit"
        n63 = property class="VI"() -> ("FP.State"=w210:T1)  [unwired: 2 in, 2 out]
        n64 = property class="App"() -> ("App.Kind"=w216:T2)  [unwired: 2 in, 2 out]
        n65 = control-ref of="Current VI Reference"() -> (w211:refnum<vi>)
        n66 = Equal?(x=w210, y=T1."Closed" ("Front Panel Window:State")) -> (x = y?=w208:bool)
        n67 = Equal?(x=w216, y=T2."Run Time System" ("Application:Kind")) -> (x = y?=w214:bool)
        n68 = Or(x=w208, y=w214) -> (x .or. y?=w212:bool)
        n69 = Bundle By Name(cluster=w213, "Core.Current VI Reference"=w211, "Core.Close Panel on Exit?"=w212) -> (w218:T6)
        n70 = call <vilib>:"Add State(s) to Queue__JKI_lib_State_Machine.vi"("State(s) in (\"\")"=w220) -> ("States Out"=w219:string)  [unwired: 14 in]
      }
      frame "Exit" {
        # "#CSM \"Exit\"\nCase for exiting the loop. No errors that occur here will be handled."
        n71 = call <vilib>:"Add State(s) to Queue__JKI_lib_State_Machine.vi"("State(s) in (\"\")"=w227) -> ("States Out"=w226:string)  [unwired: 14 in]
      }
      frame "---------- Data ----------" {
        # "#CSM \"Category Seperator\"\nDo not put any code in this frame."
        n72 = call <vilib>:"Add State(s) to Queue__JKI_lib_State_Machine.vi"("State(s) in (\"\")"=w233) -> ("States Out"=w232:string)  [unwired: 14 in]
      }
      frame "Data: Initialize" {
        w235 = "//准备开始测试\nReset Internal Status -@FlowCtrl //重置内部状态\n\n//测试过程\nReport TotalTime  -@ServoTest //统计返回总时间\n\n// 测试第一个 EXP\nReport CurentExpName >> abc.exp -@ ServoTestr \n\n// DIO 控制 根据需要看是否保留\n//DIOControl >> ${expname} -@ MAL_DIOCtrl //DIO控制\n\n//私服测试过程\nReport CurrentExpName >> abc.exp -@ServoTest \n解析EXP文件 >> abc.exp -@ServoTest \n硬件准备 -@ServoTest \nReport Ready -@ServoTest\n返回准备完毕状态 -@FlowCtrl\n等待二次确认 -@FlowCtrl\nReport CurentStatus >> 正在测试 -@FlowCtrl\n测试过程 -@ServoTest\n修改新数据生成标志 -@FlowCtrl\n关闭硬件 -@ServoTest\n\n// DIO 控制 根据需要看是否保留\n//DIOReset >> ${expname} -@ MAL_DIOCtrl //DIO重置\n\nReport teststatus >> 测试结束 -@FlowCtrl\nReport sjcjstop >> True  -@FlowCtrl"  # Sequence
        w237 = T5 {"Current VI Reference"=refnum, "Close Panel on Exit?"=FALSE}  # Core
        w238 = TRUE  # Your Boolean data
        # "do not delete - used by framework"
        # "Expand Bundle to add new data elements to shift register data."
        # "Data names and types of shift register data are defined by this bundle."
        # "#CSM \"Data: Initialize\"\nInitialize the shift-register data, here.\n(data names are defined by what you wire into the bundle function)"
        n73 = Bundle("Core"=w237, "Your Boolean data"=w238, "Sequence"=w235) -> (w240:T6)  [unwired: 1 in]
        n74 = call <vilib>:"Add State(s) to Queue__JKI_lib_State_Machine.vi"("State(s) in (\"\")"=w242) -> ("States Out"=w241:string)  [unwired: 14 in]
      }
      frame "Data: Cleanup" {
        # "#CSM \"Data: Cleanup\"\nCleanup any data and references, here.\n(this is called automatically, by the Macro: Exit)"
        n75 = Unbundle By Name(w245) -> ("Core.Current VI Reference"=w248:refnum<vi>)
        n76 = Close Reference(reference=w248, error in (no error)=w247) -> (error out=w246:errorcluster)
        n77 = call <vilib>:"Add State(s) to Queue__JKI_lib_State_Machine.vi"("State(s) in (\"\")"=w250) -> ("States Out"=w249:string)  [unwired: 14 in]
      }
      frame "---------- Events ----------" {
        # "#CSM \"Category Seperator\"\nDo not put any code in this frame."
        n78 = call <vilib>:"Add State(s) to Queue__JKI_lib_State_Machine.vi"("State(s) in (\"\")"=w256) -> ("States Out"=w255:string)  [unwired: 14 in]
      }
      frame "Events: Register" {
        # "#CSM \"Events: Register\"\nRegister user event. New Message Event is registered to break CSM waiting in event structure by default."
        # "#CSM Register New Message Event\nRegister message event to break Waiting in Event structure."
        n79 = call <userlib>:"CSM - Get New State Notifier Event.vi"("Name (\"\" to Use UUID)"=w261) -> ("error out"=w259:errorcluster, "New State Notifier Event"=w260:refnum<user-event>)  [unwired: 9 in]
        n80 = register-events(error in=w259, w260) -> (reference out=w262:refnum<event-registration>, error out=w258:errorcluster)  [unwired: 1 in]
      }
      frame "Events: Unregister" {
        # "#CSM \"Events: Unregister\"\nUnregister user event."
        n81 = Unregister For Events(event registration refnum=w266, error in=w270) -> (error out=w267:errorcluster)
      }
      frame "---------- UI ----------" {
        # "#CSM \"Category Seperator\"\nDo not put any code in this frame."
        n82 = call <vilib>:"Add State(s) to Queue__JKI_lib_State_Machine.vi"("State(s) in (\"\")"=w276) -> ("States Out"=w275:string)  [unwired: 14 in]
      }
      frame "UI: Initialize" {
        # "#CSM \"UI: Initialize\"\nInitialize the User Interface, here.\n(this is called automatically, by the Macro: Init)"
        n83 = call <vilib>:"Add State(s) to Queue__JKI_lib_State_Machine.vi"("State(s) in (\"\")"=w282) -> ("States Out"=w281:string)  [unwired: 14 in]
      }
      frame "UI: Cursor Set" {
        # "Argument"
        # "#CSM \"UI: Cursor Set\"\nSet and Unset Cursor Busy.\n(Usage: \"UI: Cursor Set >> Busy|Idle\")"
        n84 = disable-structure shown="Default" {
          disable-tunnel: w287 -> [w293 w298]
          disable-tunnel: [w292 w298] -> w286
          disable-tunnel: w285 -> [w291 _]
          frame condition #0 (active) {
            n85 = case shown="\"Busy\"" w291 {
              tunnel: w293 -> [w295 w297]
              tunnel: [w294 w296] -> w292
              frame "Idle", Default {
                n86 = call <vilib>:"Unset Busy.vi"("error in (no error)"=w295) -> ("error out"=w294:errorcluster)  [unwired: 10 in]
              }
              frame "Busy" {
                n87 = call <vilib>:"Set Busy.vi"("error in (no error)"=w297) -> ("error out"=w296:errorcluster)  [unwired: 9 in, 1 out]
              }
            }
          }
          frame condition #1 {
          }
        }
        n88 = call <vilib>:"Add State(s) to Queue__JKI_lib_State_Machine.vi"("State(s) in (\"\")"=w290) -> ("States Out"=w289:string)  [unwired: 14 in]
      }
      frame "UI: Front Panel State" {
        # "Argument"
        # "#CSM \"UI: Front Panel State\"\nSet Front Panel Open or Closed\n(Usage: \"UI: Front Panel State >> Open|Close\")"
        n89 = Unbundle By Name(w303) -> ("Core.Current VI Reference"=w302:refnum<vi>)
        n90 = case shown="\"Minimize\", \"Minimized\"" w301 {
          tunnel: w305 -> [w313 w328 w339 w352 w365]
          tunnel: [w315 w329 w341 w354 w367] -> w304
          tunnel: w302 -> [w314 w326 w340 w353 w366]
          frame "Open", "Standard", Default {
            w308 = T1."Standard" ("State")
            n91 = property class="VI"(reference=w314, error in=w313) -> (reference out=w311:refnum<vi>, error out=w312:errorcluster, "FP.State"=w310:T1)
            n92 = Not Equal?(x=w310, y=w308) -> (x != y?=w309:bool)
            n93 = case shown="True" w309 {
              tunnel: [w319 w321] -> w315
              tunnel: w312 -> [w318 w321]
              tunnel: w311 -> [w317 _]
              tunnel: w308 -> [w316 _]
              frame True {
                n94 = invoke class="VI" method="FP.Open"(reference=w317, error in=w318, "Activate"=TRUE, "State"=w316) -> (error out=w319:errorcluster)  [unwired: 1 in, 4 out]
              }
              frame False {
              }
            }
          }
          frame "Close", "Closed" {
            n95 = property class="VI"(reference=w326, error in=w328) -> (reference out=w325:refnum<vi>, error out=w327:errorcluster, "FP.State"=w323:T1)
            n96 = Not Equal?(x=w323, y=T1."Closed" ("Front Panel Window:State")) -> (x != y?=w322:bool)
            n97 = case shown="True" w322 {
              tunnel: [w330 w333] -> w329
              tunnel: w327 -> [w330 w332]
              tunnel: w325 -> [_ w331]
              frame False {
              }
              frame True {
                n98 = invoke class="VI" method="FP.Close"(reference=w331, error in=w332) -> (error out=w333:errorcluster)  [unwired: 1 in, 2 out]
              }
            }
          }
          frame "Hidden", "Hide" {
            w334 = T1."Hidden" ("State")
            n99 = property class="VI"(reference=w340, error in=w339) -> (reference out=w337:refnum<vi>, error out=w338:errorcluster, "FP.State"=w336:T1)
            n100 = Not Equal?(x=w336, y=w334) -> (x != y?=w335:bool)
            n101 = case shown="True" w335 {
              tunnel: [w345 w346] -> w341
              tunnel: w338 -> [w344 w346]
              tunnel: w337 -> [w343 _]
              tunnel: w334 -> [w342 _]
              frame True {
                n102 = invoke class="VI" method="FP.Open"(reference=w343, error in=w344, "State"=w342) -> (error out=w345:errorcluster)  [unwired: 2 in, 4 out]
              }
              frame False {
              }
            }
          }
          frame "Minimize", "Minimized" {
            w347 = T1."Minimized" ("State")
            n103 = property class="VI"(reference=w353, error in=w352) -> (reference out=w350:refnum<vi>, error out=w351:errorcluster, "FP.State"=w349:T1)
            n104 = Not Equal?(x=w349, y=w347) -> (x != y?=w348:bool)
            n105 = case shown="False" w348 {
              tunnel: [w358 w359] -> w354
              tunnel: w351 -> [w357 w359]
              tunnel: w350 -> [w356 _]
              tunnel: w347 -> [w355 _]
              frame True {
                n106 = invoke class="VI" method="FP.Open"(reference=w356, error in=w357, "State"=w355) -> (error out=w358:errorcluster)  [unwired: 2 in, 4 out]
              }
              frame False {
              }
            }
          }
          frame "Maximize", "Maximized" {
            w360 = T1."Maximized" ("State")
            n107 = property class="VI"(reference=w366, error in=w365) -> (reference out=w363:refnum<vi>, error out=w364:errorcluster, "FP.State"=w362:T1)
            n108 = Not Equal?(x=w362, y=w360) -> (x != y?=w361:bool)
            n109 = case shown="True" w361 {
              tunnel: [w371 w372] -> w367
              tunnel: w364 -> [w370 w372]
              tunnel: w363 -> [w369 _]
              tunnel: w360 -> [w368 _]
              frame True {
                n110 = invoke class="VI" method="FP.Open"(reference=w369, error in=w370, "State"=w368) -> (error out=w371:errorcluster)  [unwired: 2 in, 4 out]
              }
              frame False {
              }
            }
          }
        }
        n111 = call <vilib>:"Add State(s) to Queue__JKI_lib_State_Machine.vi"("State(s) in (\"\")"=w307) -> ("States Out"=w306:string)  [unwired: 14 in]
      }
      frame "---------- Macro ----------" {
        # "#CSM \"Category Seperator\"\nDo not put any code in this frame."
        n112 = call <vilib>:"Add State(s) to Queue__JKI_lib_State_Machine.vi"("State(s) in (\"\")"=w378) -> ("States Out"=w377:string)  [unwired: 14 in]
      }
      frame "Macro: Initialize" {
        w381 = "Data: Initialize\nInitialize Core Data\nEvents: Register\nUI: Initialize\nUI: Front Panel State >> Open"  # Data: Initialize Initialize Core Data Events: Register UI: Initialize UI: Front Panel State >> Open
        # "#CSM \"Macro: Initialize\"\nInitialization Macro (This is called once, when the VI starts)"
        n113 = call <vilib>:"Add State(s) to Queue__JKI_lib_State_Machine.vi"("State(s) in Front (\"\")"=w381, "State(s) in (\"\")"=w385) -> ("States Out"=w384:string)  [unwired: 13 in]
      }
      frame "Macro: Exit" {
        # "#CSM \"Macro: Exit\"\nExit Macro (This is called once, when the VI exits)"
        n114 = Unbundle By Name(w395) -> ("Core.Close Panel on Exit?"=w394:bool)
        n115 = Select(t="UI: Front Panel State >> Close", s=w394, f="") -> (s? t:f=w391:string)
        n116 = call <vilib>:"Add State(s) to Queue__JKI_lib_State_Machine.vi"("State(s) in Front (\"\")"="//Exit Sub-Modules ", "State(s) in (\"\")"=w391, "State(s) at Back (\"\")"="Data: Cleanup\nEvents: Unregister\nExit") -> ("States Out"=w389:string)  [unwired: 12 in]
        n117 = call <vilib>:"Add State(s) to Queue__JKI_lib_State_Machine.vi"("State(s) in Front (\"\")"=w389, "State(s) in (\"\")"=w398) -> ("States Out"=w397:string)  [unwired: 13 in]
      }
      frame "---------- API ----------" {
        # "#CSM \"Category Seperator\"\nDo not put any code in this frame."
      }
      frame "API: API1" {
        # "#CSM >> Source CSM >>\nIf you need to tell who triggered this state , use this string. If it's this case itself, this string is \"\"."
        # "#CSM >> Arguments >>\nDeal with the parameter if any"
        # "#CSM Response\nConnect this to return the response of your API"
        # "#CSM API Example\nCopy/Rename this case for your own API"
      }
      frame "API: API2" {
        # "#CSM API Example\nCopy/Rename this case for your own API"
      }
      frame "---------- Internal ----------" {
        # "#CSM \"Category Seperator\"\nDo not put any code in this frame."
        n118 = call <vilib>:"Add State(s) to Queue__JKI_lib_State_Machine.vi"("State(s) in (\"\")"=w419) -> ("States Out"=w418:string)  [unwired: 14 in]
      }
      frame "Internal: action1" {
        # "#CSM \"Internal State\"\nThis category is used for holding internal states"
        n119 = call <vilib>:"Add State(s) to Queue__JKI_lib_State_Machine.vi"("State(s) in (\"\")"=w425) -> ("States Out"=w424:string)  [unwired: 14 in]
      }
      frame "Internal: action2" {
        # "#CSM \"Internal State\"\nThis category is used for holding internal states"
        n120 = call <vilib>:"Add State(s) to Queue__JKI_lib_State_Machine.vi"("State(s) in (\"\")"=w431) -> ("States Out"=w430:string)  [unwired: 14 in]
      }
    }
  }
  n121 = call "ExecutionView(CSM).vi"("Name(\"\" to use uuid)"="TestStandOI" ("Name(\"\" to use uuid)")) -> ()  [unwired: 11 in]
  n122 = vi-ref "CSMStand(Lite).lvlib:ExecutionView(CSM).vi"() -> (w3:refnum<vi>)
  n123 = invoke on="Sub Panel" class="SubPnl" method="Insert VI"("VI Ref"=w3) -> (error out=w2:errorcluster)  [unwired: 3 in, 3 out]
  n124 = call <vilib>:"Clear Errors.vi"("error in (no error)"=w2) -> ()  [unwired: 5 in, 2 out]
